vi "Configure Load Function.vi"(8 "error in (no error)":errorcluster, 10 "Load Function (0:Fixed)":u16(ring) items=["Fixed", "List"], 11 "VISA resource name":refnum<visa-resource-name>) -> (0 "error out":errorcluster, 3 "VISA resource name out":refnum<visa-resource-name>)   [LabVIEW 2020, in "BK Precision 8600 Series.lvlib"]
doc: "Configures the load to operate in fixed mode or list mode. List mode allows programming a load sequence to run.\n\nFor list operation, use this vi to set to list mode after all step parameters and list operation parameters are configured and after the list file has been saved using <b>Save Recall List File.vi</b>."
uses:
  BK Precision 8600 Series.lvlib
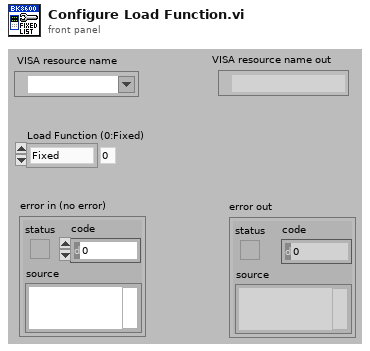
[diagram p1: front panel]
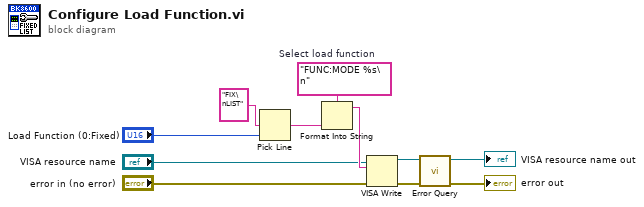
[diagram p0: block diagram]
diagram:
  w9 = "FUNC:MODE %s\n"  # Select load function
  n1 = Pick Line(multi-line string="FIX\nLIST", line index="Load Function (0:Fixed)") -> (output string=w3:string)  [unwired: 1 in]
  n2 = Format Into String(format string=w9, w3) -> (resulting string=w6:string)  [unwired: 2 in, 1 out]
  n3 = VISA Write(VISA resource name="VISA resource name", write buffer=w6, error in (no error)="error in (no error)") -> (VISA resource name out=w7:refnum<visa-resource-name>, error out=w8:errorcluster)  [unwired: 1 out]
  n4 = call "Error Query.vi"("error in (no error)"=w8, "VISA resource name"=w7) -> ("error out"=→"error out":errorcluster, "VISA resource name out"=→"VISA resource name out":refnum<visa-resource-name>)  [unwired: 6 in, 2 out]
